vi "getRefConnectionList.vi"(6 "Remote Connection":string, 8 "error in (no error)":errorcluster, 9 "new client":refnum<k5>, 10 "Enum":enum16{"read", "write", "reset", "read name"}(ring), 11 "NetworkServer in":refnum<class "NetworkServer.lvclass">) -> (0 "error out":errorcluster, 1 "client":refnum<k5>, 2 "valid?":bool, 3 "NetworkServer out":refnum<class "NetworkServer.lvclass">, 4 "Remote Connection":string)   [LabVIEW 2011, in "Hardware.lvlib" / "HWControllers.lvlib" / "NetworkServer.lvclass"]
uses:
  NetworkServer.lvclass
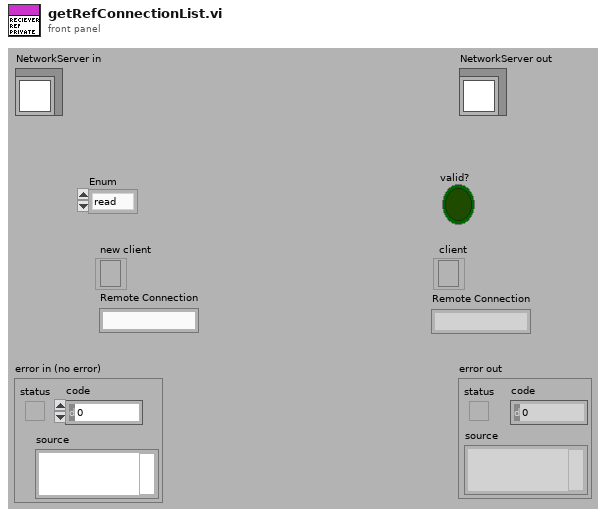
[diagram p1: front panel]
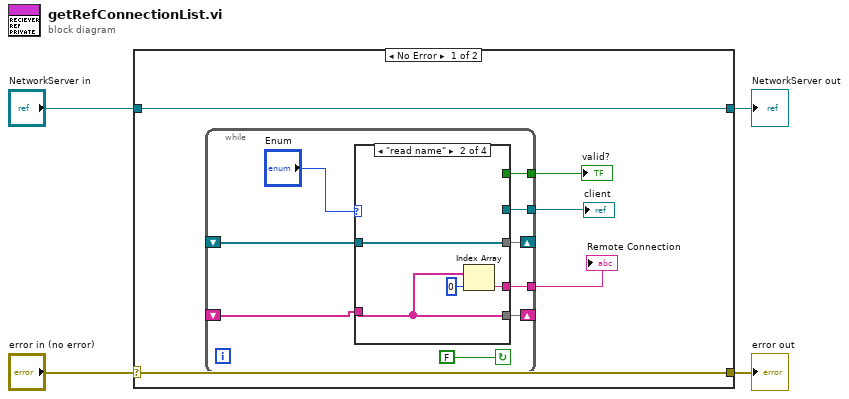
[diagram p0: block diagram]
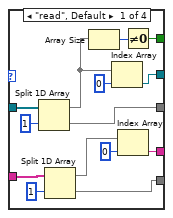
[diagram p2: hidden frame]
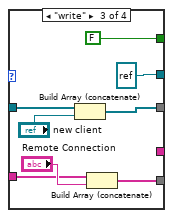
[diagram p3: hidden frame]
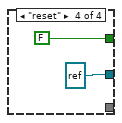
[diagram p4: hidden frame]
diagram:
  n1 = case shown="No Error" "error in (no error)" {
    selector: "error in (no error)" -> [w8 w48]
    tunnel: [w8 w48] -> w3
    tunnel: [w9 w47] -> w1
    tunnel: "NetworkServer in" -> [w9 w47]
    frame No Error {
      n2 = while {
        tunnel: [w15] -> w6
        tunnel: [w16] -> w7
        shift-left: _ -> [w17]
        shift-right: [w18] -> _
        shift-right: [w11] -> _
        shift-left: _ -> [w12]
        tunnel: [w10] -> w5
        stop <- FALSE continue-if-true
        n3 = case shown="\"read name\"" "Enum" {
          tunnel: [w30 w34 w44 _] -> w18
          tunnel: w17 -> [w32 w34 w43 _]
          tunnel: [w27 _ refnum<k5> refnum ("empty") refnum<k5> refnum ("empty")] -> w16
          tunnel: [w25 _ FALSE FALSE] -> w15
          tunnel: w12 -> [w21 w33 w38 _]
          tunnel: [w20 w33 w37 _] -> w11
          tunnel: [w19 w35 _ _] -> w10
          frame "read", Default {
            n4 = Split 1D Array(array=w32, index=1) -> (first subarray=w28:refnum<k5>[], second subarray=w30:refnum<k5>[])
            n5 = Split 1D Array(array=w21, index=1) -> (first subarray=w22:string[], second subarray=w20:string[])
            n6 = Array Size(array=w28) -> (size(s)=w26:i32)
            n7 = Index Array(array=w28, index=0) -> (element=w27:refnum<k5>)
            n8 = Index Array(array=w22, index=0) -> (element=w19:string)
            n9 = Not Equal To 0?(x=w26) -> (x != 0?=w25:bool)
          }
          frame "read name" {
            n10 = Index Array(array=w33, index=0) -> (element=w35:string)
          }
          frame "write" {
            n11 = Build Array (concatenate)(w43, "new client") -> (w44:refnum<k5>[])
            n12 = Build Array (concatenate)(w38, "Remote Connection") -> (w37:string[])
          }
          frame "reset" {
          }
        }
      }
      "client" <- w7
      "valid?" <- w6
      "Remote Connection" <- w5
    }
    frame Error {
    }
  }
  "error out" <- w3
  "NetworkServer out" <- w1
